vi "Validate the version.vi"(0 "Old Version":string[](array[string]), 5 "New Version":string[](array[string]), 11 "error in (no error)":errorcluster) -> (4 "Version Out":string[](array[string]), 15 "error out":errorcluster)   [LabVIEW 2021, in "Packager Helpers.lvlib"]
uses:
  Packager Helpers.lvlib
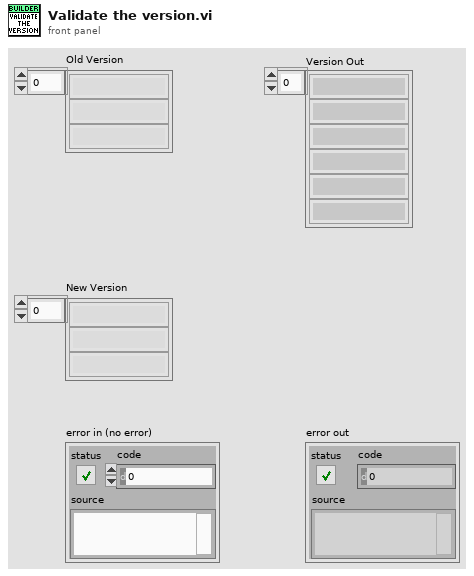
[diagram p1: front panel]
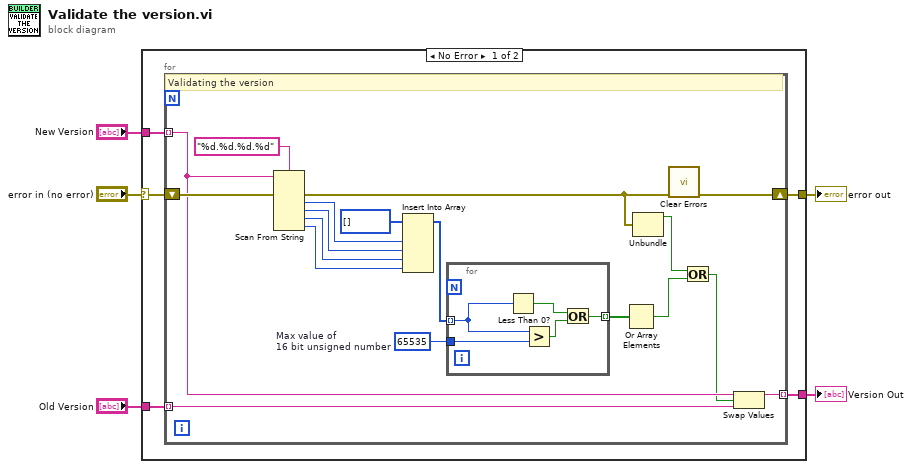
[diagram p0: block diagram]
diagram:
  n1 = case shown="No Error" "error in (no error)" {
    selector: "error in (no error)" -> [w9 w34]
    tunnel: "New Version" -> [w10 _]
    tunnel: [w8 w34] -> w3
    tunnel: [w7 _] -> w2
    tunnel: "Old Version" -> [w6 _]
    frame No Error {
      n2 = for {
        tunnel: w10 -> [w23] mode=indexing
        tunnel: [w22] -> w7 mode=indexing
        shift-right: [w25] -> w8
        shift-left: w9 -> [w28]
        tunnel: w6 -> [w24] mode=indexing
        w11 = 65535  # Max value of 16 bit unsigned number
        # "Validating the version"
        n3 = Scan From String(format string="%d.%d.%d.%d", input string=w23, error in=w28) -> (error out=w26:errorcluster, output 1=w19:i32, output 2=w18:i32, output 3=w17:i32, output 4=w16:i32)  [unwired: 5 in, 2 out]
        n4 = Insert Into Array(array=i32[] [], new element #1=w19, new element #2=w18, new element #3=w17, new element #4=w16) -> (w14:i32[])  [unwired: 1 in]
        n5 = for {
          tunnel: w14 -> [w33] mode=indexing
          tunnel: [w30] -> w13 mode=indexing
          tunnel: w11 -> [w29]
          n6 = Less Than 0?(x=w33) -> (x < 0?=w32:bool)
          n7 = Greater?(x=w33, y=w29) -> (0:w31:bool)
          n8 = Or(x=w32, y=w31) -> (x .or. y?=w30:bool)
        }
        n9 = Or Array Elements(Boolean array=w13) -> (logical OR=w12:bool)
        n10 = Unbundle(w26) -> ("status"=w21:bool)  [unwired: 2 out]
        n11 = call <vilib>:"Clear Errors.vi"("error in (no error)"=w26) -> ("error out"=w25:errorcluster)  [unwired: 5 in, 1 out]
        n12 = Or(x=w21, y=w12) -> (x .or. y?=w20:bool)
        n13 = Swap Values(12:w23, 13:w20, 14:w24) -> (1:w22:string)  [unwired: 1 out]
      }
    }
    frame Error {
    }
  }
  "error out" <- w3
  "Version Out" <- w2
